vi "toStateCluster.vi"(4 "state":T1, 5 "Anything":variant) -> (1 "output cluster":cluster{"Anything":variant, "state":T1})   [LabVIEW 2009]
uses:
  typedefs/main_States.ctl
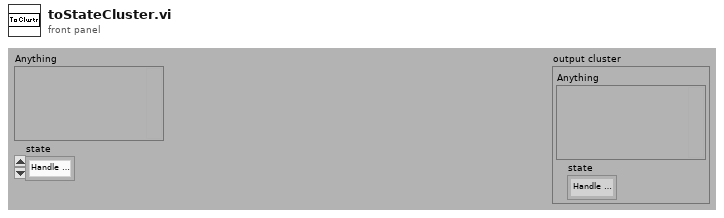
[diagram p1: front panel]
types:
  T1 = typedef "main_States.ctl" = enum16{"Handle FP Events", "Same as Scan Axis", "Exit", "Axis Start", "Open Tools", "Update Stop Position", "Start Scan", "Axis Stop", "Initialize Scanner", "Abort", "Connect Serial Port", "Initialize", "Export", "Import"}
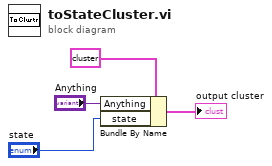
[diagram p0: block diagram]
diagram:
  n1 = Bundle By Name(cluster=cluster{"Anything":variant, "state":T1} {"Anything"=variant, "state"=enum."Handle FP Events"} ("element"), "Anything"="Anything", "state"="state") -> (→"output cluster":cluster{"Anything":variant, "state":T1})
